vi "zad2.vi"() -> ()   [LabVIEW 2017]
uses:
  <vilib>/Utility/file.llb/Read Delimited Spreadsheet (string).vi
panel:
  out "Waveform Graph":dbl[][](graph)
  out "number":dbl[][](array[numeric])
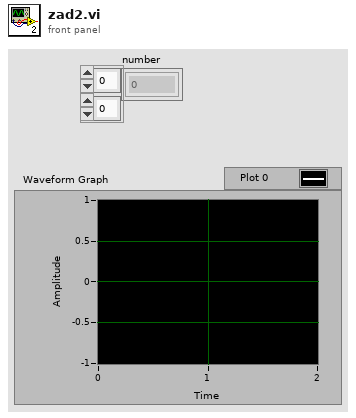
[diagram p1: front panel]
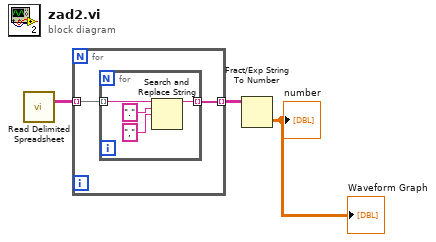
[diagram p0: block diagram]
diagram:
  n1 = call-poly <vilib>:"Read Delimited Spreadsheet.vi"() -> ("all rows"=w3:string[][])  [unwired: 10 in, 5 out]
  n2 = for {
    tunnel: w3 -> [w5] mode=indexing
    tunnel: [w4] -> w2 mode=indexing
    n3 = for {
      tunnel: w5 -> [w9] mode=indexing
      tunnel: [w6] -> w4 mode=indexing
      n4 = Search and Replace String(input string=w9, search string=".", replace string="," ("replace string (\"\")")) -> (result string=w6:string)  [unwired: 5 in, 3 out]
    }
  }
  n5 = Fract/Exp String To Number(string=w2) -> (number=→"number" →"Waveform Graph":dbl[][])  [unwired: 3 in, 1 out]
